vi "Welding_and_ActuatorSetup.vi"(0 "TCP connection IN":refnum<k5>, 5 "Number of second to wait":i32, 7 "SC_7":string, 9 "ACPC_8":string, 11 "Error In":errorcluster) -> (2 "Weld Status":bool, 3 "Absolute distance in mm":dbl, 4 "TCP connection OUT":refnum<k5>, 6 "Absolute distance in inch":dbl, 8 "Prepart contact in mm":dbl, 10 "Prepart contact in inch":dbl, 12 "SC_Params_Length":i32, 14 "AC_PC_Params_Length":i32, 15 "Error Out":errorcluster)   [LabVIEW 2017]
uses:
  Global_Variable_Status_Indicator.vi
panel:
  # "ACTUATOR SETUP : FIND PART CONTACT"
  # "Data frame structure"
  # "Command(32bit) + Size of Structure(32bit)+Parameters"
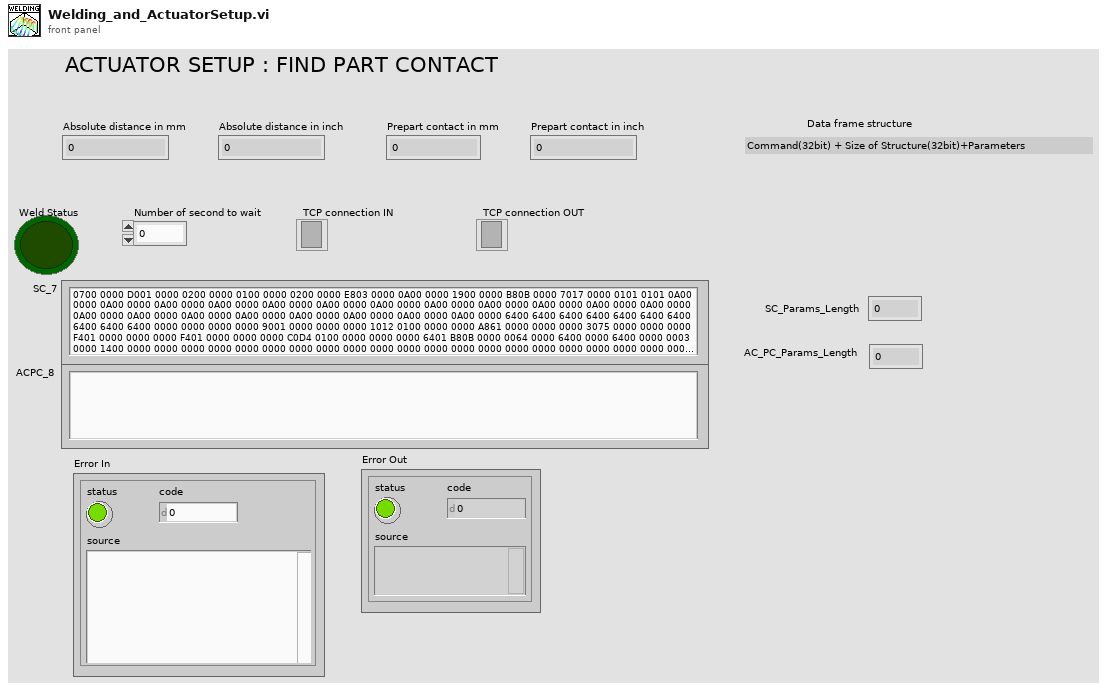
[diagram p1: front panel]
types:
  T1 = enum16{"big-endian, network order", "native, host order", "little-endian"}
  T2 = enum16{"Standard", "Buffered", "CRLF", "Immediate"}
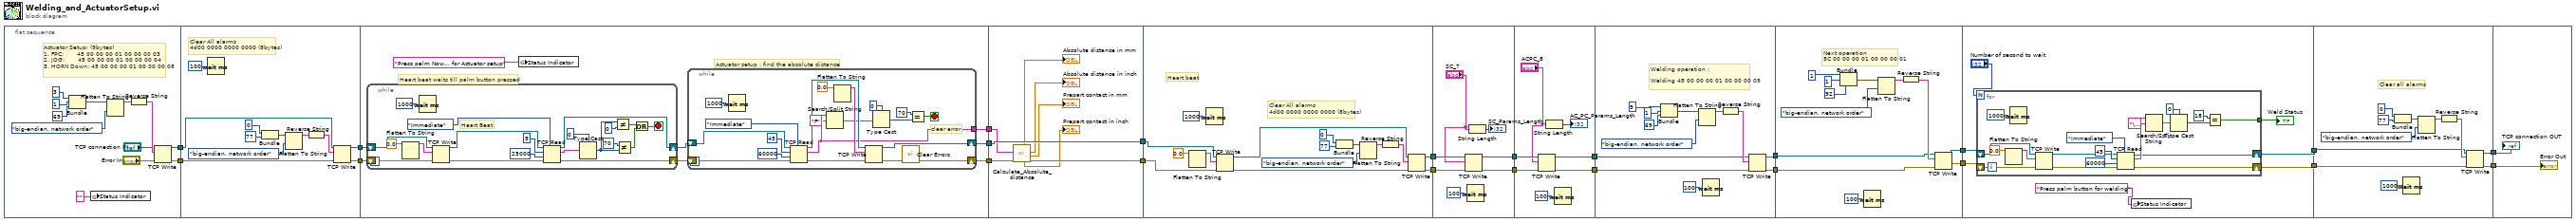
[diagram p0: block diagram]
diagram:
  n1 = flat-sequence {
    tunnel: [w33] -> w18
    tunnel: [w32] -> w16
    tunnel: w18 -> [w39]
    tunnel: [w37] -> w17
    tunnel: w16 -> [w38]
    tunnel: [w36] -> w15
    tunnel: w17 -> [w54]
    tunnel: w15 -> [w53]
    tunnel: [w52] -> w23
    tunnel: [w51] -> w22
    tunnel: [w48] -> w21
    tunnel: w23 -> [w102]
    tunnel: w22 -> [w101]
    tunnel: w21 -> [w99]
    tunnel: [w100] -> w20
    tunnel: [w102] -> w19
    tunnel: w20 -> [w117]
    tunnel: w19 -> [w116]
    tunnel: [w104] -> w4
    tunnel: [w103] -> w3
    tunnel: w4 -> [w123]
    tunnel: [w121] -> w8
    tunnel: w3 -> [w122]
    tunnel: [w122] -> w7
    tunnel: w8 -> [w129]
    tunnel: w7 -> [w128]
    tunnel: [w128] -> w2
    tunnel: [w126] -> w1
    tunnel: w2 -> [w141]
    tunnel: [w140] -> w10
    tunnel: [w139] -> w9
    tunnel: w1 -> [w130]
    tunnel: [w143] -> w12
    tunnel: [w144] -> w11
    tunnel: w10 -> [w146]
    tunnel: w9 -> [w145]
    tunnel: w12 -> [w160]
    tunnel: w11 -> [w159]
    tunnel: [w155] -> w14
    tunnel: [w156] -> w13
    tunnel: w14 -> [w184]
    tunnel: w13 -> [w183]
    tunnel: [w182] -> w6
    tunnel: [w181] -> w5
    tunnel: w6 -> [w192]
    tunnel: w5 -> [w191]
    frame #0 {
      # "Actuator Setup: (9bytes)\n1. FPC:       45 00 00 00 01 00 00 00 03\n2. JOG:       45 00 00 00 01 00 00 00 04\n3. HORN Down: 45 00 00 00 01 00 00 00 08"
      n2 = Bundle(i8 3, 1, 69) -> (w29:cluster{i8, i32, i32})  [unwired: 1 in]
      n3 = global write "Global_Variable_Status_Indicator.vi" "Status Indicator"("" ("String")) -> ()
      n4 = Flatten To String(anything=w29, byte order (0:big-endian, network order)=T1."big-endian, network order") -> (data string=w35:string)  [unwired: 2 in, 2 out]
      n5 = Reverse String(1:w35) -> (0:w34:string)
      n6 = TCP Write(connection ID="TCP connection IN", data in=w34, error in (no error)="Error In") -> (connection ID out=w33:refnum<k5>, error out=w32:errorcluster)  [unwired: 1 in, 1 out]
    }
    frame #1 {
      # "Clear All alarms\n4d00 0000 0000 0000 (8bytes)"
      n7 = Wait (ms)(milliseconds to wait=u32 100) -> ()  [unwired: 1 out]
      n8 = Bundle(0, 77) -> (w46:cluster{i32, i32})  [unwired: 1 in]
      n9 = Flatten To String(anything=w46, byte order (0:big-endian, network order)=T1."big-endian, network order") -> (data string=w45:string)  [unwired: 2 in, 2 out]
      n10 = Reverse String(1:w45) -> (0:w41:string)
      n11 = TCP Write(connection ID=w39, data in=w41, error in (no error)=w38) -> (connection ID out=w37:refnum<k5>, error out=w36:errorcluster)  [unwired: 1 in, 1 out]
    }
    frame #2 {
      # "Actuator setup : find the absolute distance"
      # "Heart beat waits till palm button pressed"
      n12 = while {
        shift-right: [w72] -> w50
        shift-left: w54 -> [w74]
        shift-right: [w71] -> w49
        shift-left: w53 -> [w73]
        stop <- w59 stop-if-true
        # "Heart Beat"
        n13 = Flatten To String(anything=0.0) -> (data string=w69:string)  [unwired: 3 in, 2 out]
        n14 = Wait (ms)(milliseconds to wait=u32 1000) -> ()  [unwired: 1 out]
        n15 = TCP Write(connection ID=w74, data in=w69, error in (no error)=w73) -> (connection ID out=w68:refnum<k5>, error out=w67:errorcluster)  [unwired: 1 in, 1 out]
        n16 = TCP Read(connection ID=w68, bytes to read=9, error in (no error)=w67, 7:T2."Immediate" ("mode (standard)"), 9:25000 ("timeout ms (25000)")) -> (connection ID out=w72:refnum<k5>, data out=w62:string, error out=w71:errorcluster)
        n17 = Type Cast(type=u8 0, x=w62) -> (*(type *) &x=w55:u8)
        n18 = Not Equal?(x=w55, y=u8 0) -> (x != y?=w57:bool)
        n19 = Not Equal?(x=u8 70, y=w55) -> (x != y?=w58:bool)
        n20 = Or(x=w57, y=w58) -> (x .or. y?=w59:bool)
      }
      n21 = global write "Global_Variable_Status_Indicator.vi" "Status Indicator"("Press palm Now... for Actuator setup" ("Status indicator")) -> ()
      n22 = while {
        tunnel: [w77] -> w48
        shift-right: [w82] -> w52
        shift-left: w50 -> [w94]
        shift-right: [w81] -> w51
        shift-left: w49 -> [w93]
        stop <- w88 stop-if-true
        # "clear error"
        n23 = Wait (ms)(milliseconds to wait=u32 1000) -> ()  [unwired: 1 out]
        n24 = TCP Read(connection ID=w94, bytes to read=45, error in (no error)=w93, 7:T2."Immediate" ("mode (standard)"), 9:60000 ("timeout ms (25000)")) -> (connection ID out=w85:refnum<k5>, data out=w77:string, error out=w84:errorcluster)
        n25 = Search/Split String(string=w77, search string/char (-)="F") -> (match + rest of string=w75:string)  [unwired: 1 in, 2 out]
        n26 = Flatten To String(anything=0.0) -> (data string=w86:string)  [unwired: 3 in, 2 out]
        n27 = TCP Write(connection ID=w85, data in=w86, error in (no error)=w84) -> (connection ID out=w82:refnum<k5>, error out=w83:errorcluster)  [unwired: 1 in, 1 out]
        n28 = Type Cast(type=u8 0, x=w75) -> (*(type *) &x=w80:u8)
        n29 = call <vilib>:"Clear Errors.vi"("error in (no error)"=w83) -> ("error out"=w81:errorcluster)  [unwired: 5 in, 1 out]
        n30 = Equal?(x=u8 70, y=w80) -> (x = y?=w88:bool)
      }
    }
    frame #3 {
      n31 = call "Calculate_Absolute_distance.vi"("Error In"=w101, "data in"=w99) -> ("Error Out"=w100:errorcluster, "Prepart contact in mm"=→"Prepart contact in mm":dbl, "Absolute distance in inch"=→"Absolute distance in inch":dbl, "Prepart contact in inch"=→"Prepart contact in inch":dbl, "Absolute distance in mm"=→"Absolute distance in mm":dbl)  [unwired: 4 in, 1 out]
    }
    frame #4 {
      # "Clear All alarms\n4d00 0000 0000 0000 (8bytes)"
      # "Heart beat"
      n32 = Flatten To String(anything=0.0) -> (data string=w111:string)  [unwired: 3 in, 2 out]
      n33 = Wait (ms)(milliseconds to wait=u32 1000) -> ()  [unwired: 1 out]
      n34 = TCP Write(connection ID=w116, data in=w111, error in (no error)=w117) -> (connection ID out=w115:refnum<k5>, error out=w114:errorcluster)  [unwired: 1 in, 1 out]
      n35 = Bundle(0, 77) -> (w110:cluster{i32, i32})  [unwired: 1 in]
      n36 = Flatten To String(anything=w110, byte order (0:big-endian, network order)=T1."big-endian, network order") -> (data string=w109:string)  [unwired: 2 in, 2 out]
      n37 = Reverse String(1:w109) -> (0:w105:string)
      n38 = TCP Write(connection ID=w115, data in=w105, error in (no error)=w114) -> (connection ID out=w104:refnum<k5>, error out=w103:errorcluster)  [unwired: 1 in, 1 out]
    }
    frame #5 {
      n39 = TCP Write(connection ID=w123, data in="SC_7") -> (connection ID out=w121:refnum<k5>)  [unwired: 2 in, 2 out]
      n40 = Wait (ms)(milliseconds to wait=u32 100) -> ()  [unwired: 1 out]
      n41 = String Length(string="SC_7") -> (length=→"SC_Params_Length":i32)
    }
    frame #6 {
      n42 = TCP Write(connection ID=w129, data in="ACPC_8") -> (connection ID out=w126:refnum<k5>)  [unwired: 2 in, 2 out]
      n43 = String Length(string="ACPC_8") -> (length=→"AC_PC_Params_Length":i32)
      n44 = Wait (ms)(milliseconds to wait=u32 100) -> ()  [unwired: 1 out]
    }
    frame #7 {
      # "Welding operation :\n\nWelding 45 00 00 00 01 00 00 00 09"
      n45 = Bundle(i8 9, 1, 69) -> (w134:cluster{i8, i32, i32})  [unwired: 1 in]
      n46 = Flatten To String(anything=w134, byte order (0:big-endian, network order)=T1."big-endian, network order") -> (data string=w137:string)  [unwired: 2 in, 2 out]
      n47 = Wait (ms)(milliseconds to wait=u32 100) -> ()  [unwired: 1 out]
      n48 = Reverse String(1:w137) -> (0:w131:string)
      n49 = TCP Write(connection ID=w130, data in=w131, error in (no error)=w141) -> (connection ID out=w139:refnum<k5>, error out=w140:errorcluster)  [unwired: 1 in, 1 out]
    }
    frame #8 {
      # "Next operation\n5C 00 00 00 01 00 00 00 01"
      n50 = Bundle(i8 1, 1, 92) -> (w152:cluster{i8, i32, i32})  [unwired: 1 in]
      n51 = Wait (ms)(milliseconds to wait=u32 100) -> ()  [unwired: 1 out]
      n52 = Flatten To String(anything=w152, byte order (0:big-endian, network order)=T1."big-endian, network order") -> (data string=w151:string)  [unwired: 2 in, 2 out]
      n53 = Reverse String(1:w151) -> (0:w153:string)
      n54 = TCP Write(connection ID=w145, data in=w153, error in (no error)=w146) -> (connection ID out=w143:refnum<k5>, error out=w144:errorcluster)  [unwired: 1 in, 1 out]
    }
    frame #9 {
      n55 = for {
        N: "Number of second to wait" -> [_]
        shift-right: [w165] -> w156
        shift-left: w160 -> [w179]
        shift-right: [w164] -> w155
        shift-left: w159 -> [w178]
        tunnel: [w161] -> w154
        n56 = Flatten To String(anything=0.0) -> (data string=w176:string)  [unwired: 3 in, 2 out]
        n57 = Wait (ms)(milliseconds to wait=u32 1000) -> ()  [unwired: 1 out]
        n58 = TCP Write(connection ID=w179, data in=w176, error in (no error)=w178) -> (connection ID out=w163:refnum<k5>, error out=w162:errorcluster)  [unwired: 1 in, 1 out]
        n59 = TCP Read(connection ID=w163, bytes to read=45, error in (no error)=w162, 7:T2."Immediate" ("mode (standard)"), 9:60000 ("timeout ms (25000)")) -> (connection ID out=w165:refnum<k5>, data out=w170:string, error out=w164:errorcluster)
        n60 = Search/Split String(string=w170, search string/char (-)="\u0012") -> (match + rest of string=w166:string)  [unwired: 1 in, 2 out]
        n61 = Type Cast(type=u8 0, x=w166) -> (*(type *) &x=w169:u8)
        n62 = Equal?(x=u8 18, y=w169) -> (x = y?=w161:bool)
      }
      "Weld Status" <- w154
      n63 = global write "Global_Variable_Status_Indicator.vi" "Status Indicator"("Press palm button for welding" ("Status indicator")) -> ()
    }
    frame #10 {
      # "Clear all alarms"
      n64 = Bundle(0, 77) -> (w190:cluster{i32, i32})  [unwired: 1 in]
      n65 = Wait (ms)(milliseconds to wait=u32 1000) -> ()  [unwired: 1 out]
      n66 = Flatten To String(anything=w190, byte order (0:big-endian, network order)=T1."big-endian, network order") -> (data string=w189:string)  [unwired: 2 in, 2 out]
      n67 = Reverse String(1:w189) -> (0:w185:string)
      n68 = TCP Write(connection ID=w183, data in=w185, error in (no error)=w184) -> (connection ID out=w181:refnum<k5>, error out=w182:errorcluster)  [unwired: 1 in, 1 out]
    }
    frame #11 {
      "Error Out" <- w192
      "TCP connection OUT" <- w191
    }
  }
